vi "SVD ReadVT_SGL.vi"(8 "error in (no error)":errorcluster, 10 "Dst in":sgl[][](array[numeric]), 11 "SVD in":refnum<class "SVD.lvclass">) -> (0 "error out":errorcluster, 2 "Dst  out":sgl[][](array[numeric]), 3 "SVD out":refnum<class "SVD.lvclass">)   [LabVIEW 2020, in "OpenLvVision_OpenCv.lvlib" / "SVD.lvclass"]
doc: "Copies the W mat form the object."
uses:
  SVD.lvclass
  C:/Users/lukas/Downloads/OpenLvVision_OpenCv/SourceCode/LabView/OpenLvVision_OpenCv/_LvHelpers/EdvrObject/EdvrObject.lvclass
  TypeDef/LvDatatype.ctl
  _LvHelpers/EdvrObject/EdvrObject.lvclass/EdvrObject.ctl
  _LvHelpers/MatHandling/WriteSize/WriteSizeMat_2DArray_SGL.vi
  _LvHelpers/MatHandling/RegisterMat/RegisterMat_Array2D-SGL.vi
  <vilib>/Utility/error.llb/Error Cluster From Error Code.vi
  _LvHelpers/MatHandling/UnregisterMat/UnregisterMat_2DArray-SGL.vi
  <vilib>/ErrorRing/Error Ring.xnode
  _LvHelpers/EdvrObject/EdvrObject.lvclass
  OpenLvVision_OpenCv.lvlib
  Dlls/OlvOpenCvWrapper.dll
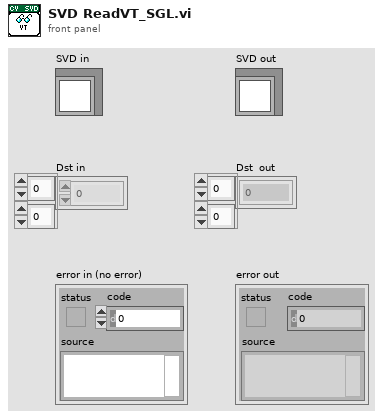
[diagram p1: front panel]
types:
  T1 = typedef "OpenLvVision_OpenCv.lvlib/LvDatatype.ctl" = enum32{"Undefined", "U8", "I8", "U16", "I16", "U32_Color", "I32", "U64_Color", "I64", "SGL", "DBL", "Complex SGL", "Complex DBL", "Array 1D U8", "Array 1D I8", "Array 1D U16", "Array 1D I16", "Array 1D U32_Color", "Array 1D I32", "Array 1D U64_Color", "Array 1D I64", "Array 1D SGL", "Array 1D DBL", "Array 1D Complex SGL", "Array 1D Complex DBL", "Array 2D U8", "Array 2D I8", "Array 2D U16", "Array 2D I16", "Array 2D U32", "Array 2D U32_Color", "Array 2D I32", "Array 2D U64", "Array 2D U64_Color", "Array 2D I64", "Array 2D SGL", "Array 2D DBL", "Array 2D Complex SGL", "Array 2D Complex DBL", "Image Mono U8", "Image Mono U16", "Image Mono I16", "Image Mono SGL", "Image Color U32", "Image Color U64", "ImageComplex Sgl", "Array1d_2dPointI32", "Array1d_2dPointSGL", "Array1d_2dPointDBL", "Array1d_3dPointI32", "Array1d_3dPointSGL", "Array1d_3dPointDBL", "Array1d_4dPointI32", "Array1d_4dPointSGL", "Array1d_4dPointDBL"}
  T2 = typedef "OpenLvVision_OpenCv.lvlib/MatInfo.ctl" = cluster{"Datatype":T1, "Height":i32, "Width":i32, "Channels":i32, "LineWidth":i32, "Null":u8}
  T3 = typedef "OpenLvVision_OpenCv.lvlib/EdvrObject.lvclass/Edvr.ctl" = refnum<data-value>
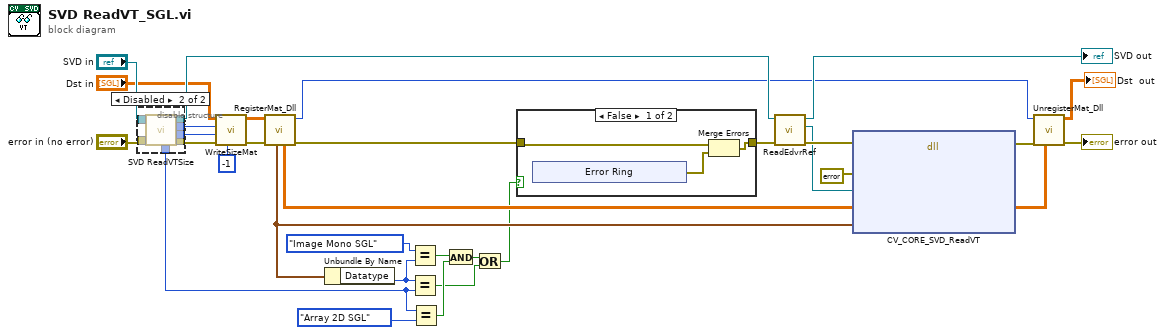
[diagram p0: block diagram]
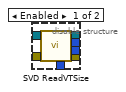
[diagram p2: hidden frame]
diagram:
  n1 = disable-structure shown="Disabled" {
    disable-tunnel: "SVD in" -> [w39 w46]
    disable-tunnel: "error in (no error)" -> [w38 w45]
    disable-tunnel: [w37 w44] -> w26
    disable-tunnel: [w36 w43] -> w18
    disable-tunnel: [w35 w42] -> w15
    disable-tunnel: [w34 w41] -> w14
    disable-tunnel: [w33 w40] -> w9
    frame Enabled {
      n2 = call "SVD ReadVTSize.vi"("error in (no error)"=w38, "SVD in"=w39) -> ("error out"=w36:errorcluster, "Rows"=w34:i32, "Cols"=w35:i32, "SVD out"=w37:refnum<class "SVD.lvclass">, "Datatype"=w33:T1)  [unwired: 5 in]
    }
    frame Disabled {
      n3 = call "SVD ReadVTSize.vi"("error in (no error)"=w45, "SVD in"=w46) -> ("error out"=w43:errorcluster, "Rows"=w41:i32, "Cols"=w42:i32, "SVD out"=w44:refnum<class "SVD.lvclass">, "Datatype"=w40:T1)  [unwired: 5 in]
    }
  }
  n4 = call-poly "WriteSizeMat.vi"("Channel"=-1, "error in"=w18, "Height"=w14, "Width"=w15, "Array in"="Dst in") -> ("error out"=w20:errorcluster, "Array out"=w19:sgl[][])  [unwired: 5 in]
  n5 = call-poly "RegisterMat_Dll.vi"("error in"=w20, "Array in"=w19) -> ("error out"=w12:errorcluster, "Image"=w21:u8, "AdressOrData"=w25:sgl[][], "Mat"=w10:T2)  [unwired: 6 in]
  n6 = Unbundle By Name(w10) -> ("Datatype"=w7:T1)
  n7 = Equal?(x=LvDatatype."Image Mono SGL" ("Datatype"), y=w7) -> (x = y?=w5:bool)
  n8 = Equal?(x=w7, y=w9) -> (x = y?=w2:bool)
  n9 = Equal?(x=w9, y=LvDatatype."Array 2D SGL" ("Datatype")) -> (x = y?=w4:bool)
  n10 = And(x=w5, y=w4) -> (x .and. y?=w3:bool)
  n11 = Or(x=w3, y=w2) -> (x .or. y?=w1:bool)
  n12 = case shown="False" w1 {
    tunnel: w12 -> [w49 w55]
    tunnel: [w47 w55] -> w11
    frame False {
      n13 = xnode "Error Ring"() -> ("error out"=w48:errorcluster)
      n14 = Merge Errors(w49, w48) -> (w47:errorcluster)
    }
    frame True {
    }
  }
  n15 = call "ReadEdvrRef.vi"("error in (no error)"=w11, "EdvrObject in"=w26) -> ("error out"=w32:errorcluster, "Edvr"=w30:T3, "EdvrObject out"=→"SVD out":refnum<class "SVD.lvclass">)  [unwired: 7 in]
  n16 = dll-call lib="C:/Users/lukas/Downloads/OpenLvVision_OpenCv/SourceCode/LabView/OpenLvVision_OpenCv/Dlls/OlvOpenCvWrapper.dll" fn="CV_CORE_SVD_ReadVT"(error in=w32, "Error"=errorcluster {"status"=FALSE, "code"=0, "source"=""} ("error out"), "edvrRef"=w30, "AddressDst"=w25, "MatInfoDst"=w10) -> (error out=w24:errorcluster, "AddressDst"=w23:sgl[][])  [unwired: 6 in, 1 out]
  n17 = call-poly "UnregisterMat_Dll.vi"("AdressOrData"=w23, "error in"=w24, "Image"=w21) -> ("error out"=→"error out":errorcluster, "Datatype"=→"Dst  out":sgl[][])  [unwired: 7 in]
